vi "createActuator.vi"(8 "error in (no error)":errorcluster, 10 "Actuator Types":T1, 11 "IActuatorFactory in":refnum<class "IActuatorFactory.lvclass">) -> (0 "error out":errorcluster, 2 "Actuator":refnum<class "IActuator.lvclass">, 3 "IActuatorFactory out":refnum<class "IActuatorFactory.lvclass">)   [LabVIEW 2015, in "IActuatorFactory.lvclass"]
uses:
  IActuatorFactory.lvclass
  IActuator/IActuator.lvclass
  Typedefs/Actuator Types.ctl
  Typedefs/FAMTTypedefs.lvlib
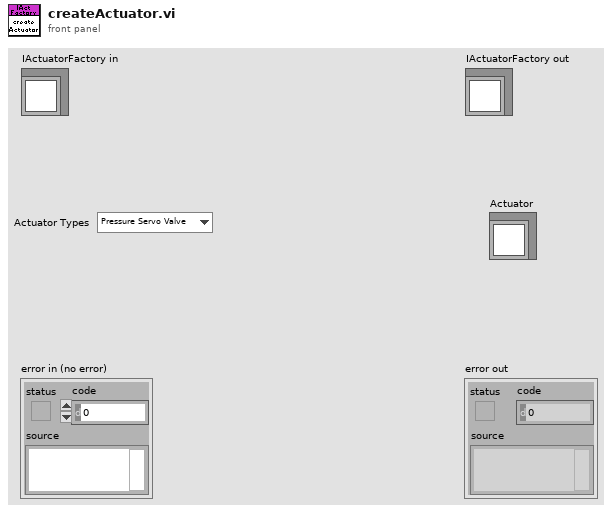
[diagram p1: front panel]
types:
  T1 = typedef "FAMTTypedefs.lvlib/Actuator Types.ctl" = enum16{"Pressure Servo Valve", "Flow Control Valve"}
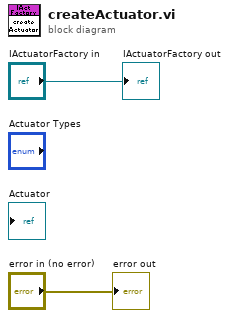
[diagram p0: block diagram]
diagram:
  "error out" <- "error in (no error)"
  "IActuatorFactory out" <- "IActuatorFactory in"
